vi "Fibonnaci.vi"() -> ()   [LabVIEW 2019]
panel:
  out "Array":u8[](array[numeric])
  in  "Numeric":i32
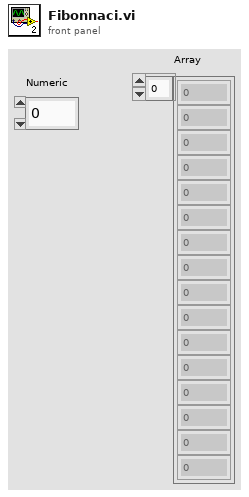
[diagram p1: front panel]
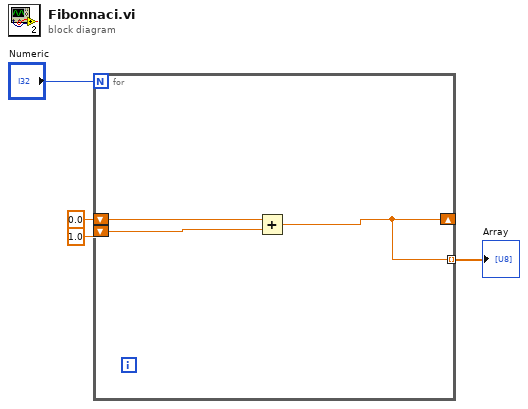
[diagram p0: block diagram]
diagram:
  n1 = for {
    N: "Numeric" -> [_]
    shift-right: [w5] -> _
    shift-left: 0.0 -> [w6]
    shift-left: 1.0 -> [w7]
    tunnel: [w5] -> w1 mode=indexing
    n2 = Add(x=w6, y=w7) -> (x+y=w5:dbl)
  }
  "Array" <- w1
